vi "SendUpstreamMessage.vi"(8 "error in (no error)":errorcluster, 10 "UpstreamMsg":refnum<class "UpstreamMsgParent.lvclass">, 11 "Message Handling in":refnum<class "Message Handling.lvclass">) -> (0 "error out":errorcluster, 3 "Message Handling out":refnum<class "Message Handling.lvclass">)   [LabVIEW 2020, in "Message Handling.lvlib" / "Message Handling.lvclass"]
uses:
  Message Handling.lvclass
  UpstreamMsg/UpstreamMsgParent/UpstreamMsgParent.lvclass
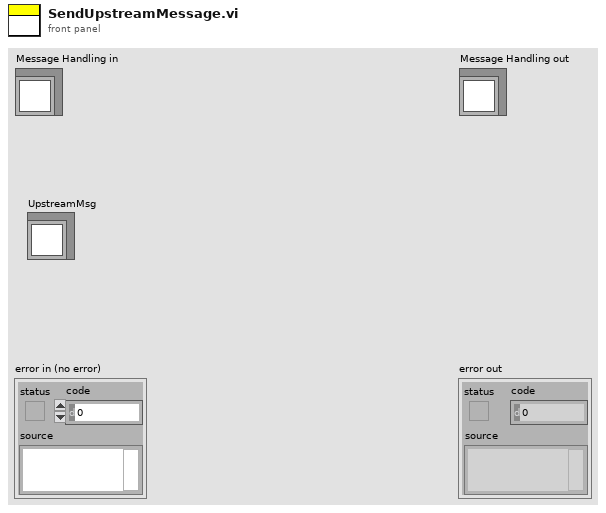
[diagram p1: front panel]
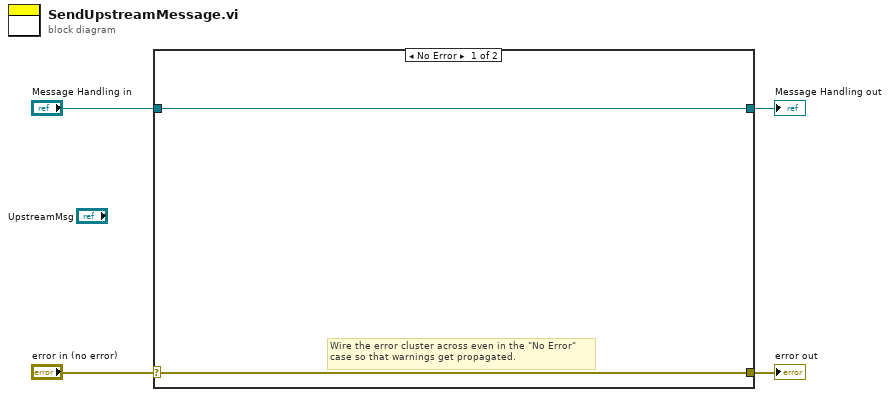
[diagram p0: block diagram]
diagram:
  n1 = case shown="No Error" "error in (no error)" {
    selector: "error in (no error)" -> [w5 w8]
    tunnel: [w5 w8] -> w3
    tunnel: [w6 w7] -> w1
    tunnel: "Message Handling in" -> [w6 w7]
    frame No Error {
      # "Wire the error cluster across even in the \"No Error\"\ncase so that warnings get propagated."
    }
    frame Error {
    }
  }
  "error out" <- w3
  "Message Handling out" <- w1
